vi "bootmode_lua.vi"(5 "LuaVIEW reference":T1) -> (15 "error out":errorcluster)   [LabVIEW 2012]
doc: "Returns the bootmode of the server application as configured in the bootstrap script. The bootmode value is intended for conditional execution of initialisation and configuration actions. The returned value reflects the value of a LabVIEW global so the mode can also be referenced from LabVIEW code. A typical use is to discriminate between \"operational\" and \"test\" modes so that the server can run with and without instrumentation.\nResults:\nstr:mode"
uses:
  luaview/typedefs/t_LuaVIEW Reference.ctl
  luaview/glb_LuaVIEW Configuration Globals.vi
  luaview/subvis/private/LuaVIEW Push (string).vi
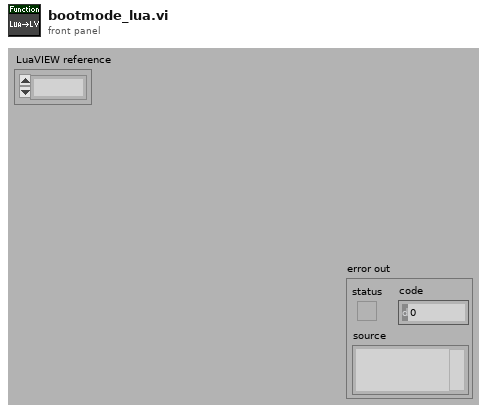
[diagram p1: front panel]
types:
  T1 = typedef "t_LuaVIEW Reference.ctl" = refnum<k1>
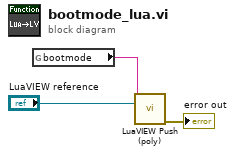
[diagram p0: block diagram]
diagram:
  n1 = global read "glb_LuaVIEW Configuration Globals.vi" "bootmode"() -> (w2:string)
  n2 = call-poly "LuaVIEW Push (poly).vi"("string"=w2, "LuaVIEW reference in"="LuaVIEW reference") -> ("error out"=→"error out":errorcluster)  [unwired: 12 in, 1 out]
